vi "Joystick_Deadband.vi"(10 "band":dbl=0.08 format="%#_13g", 11 "in":dbl) -> (3 "out":dbl)   [LabVIEW 2014]
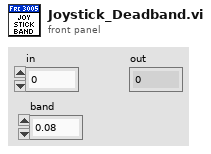
[diagram p1: front panel]
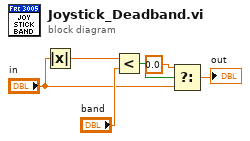
[diagram p0: block diagram]
diagram:
  n1 = Absolute Value(x="in") -> (abs(x)=w6:dbl)
  n2 = Less?(x=w6, y="band") -> (x < y?=w4:bool)
  n3 = Select(t=0.0, s=w4, f="in") -> (s? t:f=→"out":dbl)
